vi "Animate Beer.vi"(10 "Type":enum16{"Lager", "Ale", "Guiness"}(ring)=enum."Guiness", 11 "Tilt":bool) -> ()   [LabVIEW 2011]
doc: "This shows teh animation of a beer being poured"
uses:
  <vilib>/vision/NI_Vision_Development_Module.lvlib
panel:
  out "Image 2":T1(plugin-control)
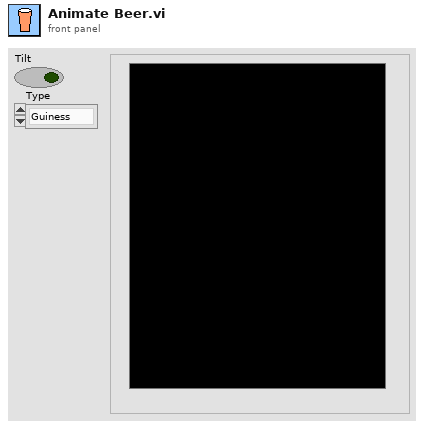
[diagram p1: front panel]
types:
  T1 = typedef "IMAQ Image.ctl" = refnum<image>
  T2 = typedef "Image Type" = u32
  T3 = cluster{"Red or Hue value":u8, "Green or Sat value":u8, "Blue or Luma or Val or Inten value":u8}
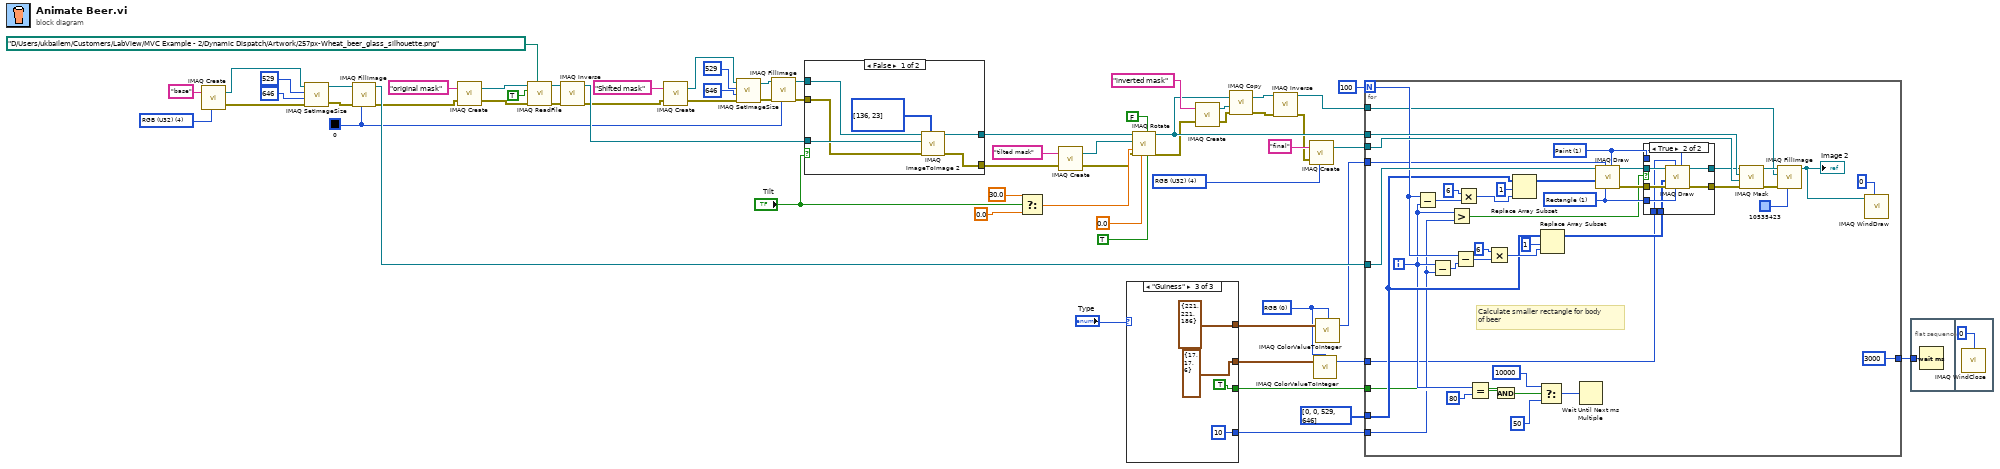
[diagram p0: block diagram]
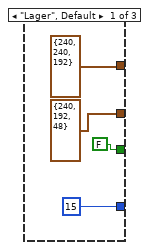
[diagram p2: hidden frame]
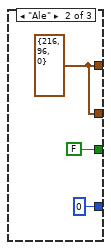
[diagram p3: hidden frame]
diagram:
  w18 = u16 0 items=["RGB", "HSL", "HSV", "HSI"] ("Color Mode")
  w16 = u32 0 ("Color Pixel Value")
  w43 = T2 4 items=["Grayscale (U8)", "Grayscale (I16)", "Grayscale (SGL)", "Complex (CSG)", "RGB (U32)", "HSL (U32)", "RGB (U64)", "Grayscale (U16)"] ("Image Type")
  w52 = T2 4 items=["Grayscale (U8)", "Grayscale (I16)", "Grayscale (SGL)", "Complex (CSG)", "RGB (U32)", "HSL (U32)", "RGB (U64)", "Grayscale (U16)"] ("Image Type")
  n1 = call "IMAQ Create"("Image Name"="base", "Image Type"=w52) -> ("New Image"=w51:T1, "error out"=w50:errorcluster)  [unwired: 3 in]
  n2 = call "IMAQ SetImageSize"("error in (no error)"=w50, "Y Resolution"=646, "X Resolution"=529, "Image"=w51) -> ("error out"=w47:errorcluster, "Image Out"=w48:T1)  [unwired: 1 in]
  n3 = call "IMAQ FillImage"("Color Pixel Value"=w16, "error in (no error)"=w47, "Image"=w48) -> ("error out"=w21:errorcluster, "Image Out"=w45:T1)  [unwired: 7 in]
  n4 = call "IMAQ Create"("Image Name"="original mask", "error in (no error)"=w21) -> ("New Image"=w62:T1, "error out"=w63:errorcluster)  [unwired: 3 in]
  n5 = call "IMAQ ReadFile"("File Path"=path "D:/Users/ukbailem/Customers/LabView/MVC Example - 2/Dynamic Dispatch/Artwork/257px-Wheat_beer_glass_silhouette.png" ("Path"), "error in (no error)"=w63, "Load Color Palette? (No)"=TRUE, "Image"=w62) -> ("error out"=w23:errorcluster, "Image Out"=w54:T1)  [unwired: 3 in, 3 out]
  n6 = call "IMAQ Inverse"("error in (no error)"=w23, "Image Src"=w54) -> ("error out"=w22:errorcluster, "Image Dst Out"=w28:T1)  [unwired: 8 in]
  n7 = call "IMAQ Create"("Image Name"="Shifted mask", "error in (no error)"=w22) -> ("New Image"=w33:T1, "error out"=w32:errorcluster)  [unwired: 3 in]
  n8 = call "IMAQ SetImageSize"("error in (no error)"=w32, "Y Resolution"=646, "X Resolution"=529, "Image"=w33) -> ("error out"=w31:errorcluster, "Image Out"=w30:T1)  [unwired: 1 in]
  n9 = call "IMAQ FillImage"("Color Pixel Value"=w16, "error in (no error)"=w31, "Image"=w30) -> ("error out"=w20:errorcluster, "Image Out"=w29:T1)  [unwired: 7 in]
  n10 = case shown="False" "Tilt" {
    tunnel: w29 -> [w70 _]
    tunnel: w28 -> [w69 w72]
    tunnel: [w68 w72] -> w27
    tunnel: w20 -> [w66 w71]
    tunnel: [w65 w71] -> w13
    frame False {
      n11 = call "IMAQ ImageToImage 2"("Offset Left/Top"=i32[] [136, 23], "error in (no error)"=w66, "Image Src (Small)"=w69, "Image Src (Large)"=w70) -> ("error out"=w65:errorcluster, "Image Dst Out"=w68:T1)  [unwired: 6 in]
    }
    frame True {
    }
  }
  n12 = Select(t=sgl 30.0 ("Angle (degrees)"), s="Tilt", f=sgl 0.0) -> (s? t:f=w38:sgl)
  n13 = call "IMAQ Create"("Image Name"="tilted mask", "error in (no error)"=w13) -> ("New Image"=w58:T1, "error out"=w3:errorcluster)  [unwired: 3 in]
  n14 = case shown="\"Guiness\"" "Type" {
    tunnel: [T3 {"Red or Hue value"=240, "Green or Sat value"=240, "Blue or Luma or Val or Inten value"=192} ("Color Value") w79 T3 {"Red or Hue value"=221, "Green or Sat value"=221, "Blue or Luma or Val or Inten value"=186} ("Color Value")] -> w24
    tunnel: [T3 {"Red or Hue value"=240, "Green or Sat value"=192, "Blue or Luma or Val or Inten value"=48} ("Color Value") w79 T3 {"Red or Hue value"=17, "Green or Sat value"=17, "Blue or Luma or Val or Inten value"=6} ("Color Value")] -> w15
    tunnel: [FALSE FALSE TRUE] -> w14
    tunnel: [15 ("y") 0 ("y") 10 ("y")] -> w7
    frame "Lager", Default {
    }
    frame "Ale" {
      w79 = T3 {"Red or Hue value"=216, "Green or Sat value"=96, "Blue or Luma or Val or Inten value"=0} ("Color Value")
    }
    frame "Guiness" {
    }
  }
  n15 = call "IMAQ Rotate"("Use Bilinear Interpolation"=TRUE, "Maintain Size"=FALSE, "Replace Value"=sgl 0.0, "error in (no error)"=w3, "Angle (degrees)"=w38, "Image Dst"=w58, "Image Src"=w27) -> ("error out"=w1:errorcluster, "Image Dst Out"=w11:T1)  [unwired: 3 in]
  n16 = call "IMAQ Create"("Image Name"="inverted mask", "error in (no error)"=w1) -> ("New Image"=w10:T1, "error out"=w2:errorcluster)  [unwired: 3 in]
  n17 = call "IMAQ Copy"("error in (no error)"=w2, "Image Dst"=w10, "Image Src"=w11) -> ("error out"=w5:errorcluster, "Image Dst Out"=w9:T1)  [unwired: 3 in]
  n18 = call "IMAQ Inverse"("error in (no error)"=w5, "Image Src"=w9) -> ("error out"=w4:errorcluster, "Image Dst Out"=w8:T1)  [unwired: 8 in]
  n19 = call "IMAQ Create"("Image Name"="final", "Image Type"=w43, "error in (no error)"=w4) -> ("New Image"=w40:T1)  [unwired: 2 in, 1 out]
  n20 = call "IMAQ ColorValueToInteger"("Color Value"=w15, "Color Mode"=w18) -> ("U32 value"=w17:u32)  [unwired: 3 in, 3 out]
  n21 = call "IMAQ ColorValueToInteger"("Color Value"=w24, "Color Mode"=w18) -> ("U32 value"=w25:u32)  [unwired: 3 in, 3 out]
  n22 = for {
    N: 100 -> [w116]
    tunnel: w45 -> [w124]
    tunnel: i32[] [0, 0, 529, 646] ("Coordinates") -> [w106]
    tunnel: w11 -> [w120]
    tunnel: w40 -> [w119]
    tunnel: w25 -> [w85]
    tunnel: w17 -> [w84]
    tunnel: w14 -> [w94]
    tunnel: w8 -> [w92]
    tunnel: w7 -> [w89]
    tunnel: [u32 3000 ("t")] -> w6
    i -> [w96]
    w110 = u16 1 items=["Frame", "Paint", "Invert Frame", "Invert Paint"] ("Draw Mode")
    w109 = u16 1 items=["Line", "Rectangle", "Oval"] ("Shape to draw")
    # "Calculate smaller rectangle for body\nof beer"
    n23 = Subtract(x=w116, y=w96) -> (x-y=w122:i32)
    n24 = Subtract(x=w96, y=w89) -> (x-y=w117:i32)
    n25 = Greater?(x=w96, y=w89) -> (0:w104:bool)
    n26 = Subtract(x=w116, y=w117) -> (x-y=w115:i32)
    n27 = Multiply(x=6, y=w122) -> (x*y=w107:i32)
    n28 = Equal?(x=w96, y=80) -> (x = y?=w100:bool)
    n29 = Multiply(x=6, y=w115) -> (x*y=w108:i32)
    n30 = And(x=w100, y=w94) -> (x .and. y?=w95:bool)
    n31 = Replace Array Subset(array=w106, new element=w107, index=1) -> (w103:i32[])
    n32 = Select(t=u32 10000, s=w95, f=u32 50 ("millisecond multiple")) -> (s? t:f=w97:u32)
    n33 = Replace Array Subset(array=w106, new element=w108, index=1) -> (w102:i32[])
    n34 = Wait Until Next ms Multiple(millisecond multiple=w97) -> ()  [unwired: 1 out]
    n35 = call "IMAQ Draw"("Draw Mode"=w110, "Shape to draw"=w109, "Pixel Color"=w85, "Coordinates"=w103, "Image Src"=w124) -> ("error out"=w114:errorcluster, "Image Dst Out"=w111:T1)  [unwired: 5 in]
    n36 = case shown="True" w104 {
      tunnel: w114 -> [w125 w134]
      tunnel: [w125 w133] -> w113
      tunnel: [w126 w132] -> w112
      tunnel: w111 -> [w126 w131]
      tunnel: w110 -> [_ w130]
      tunnel: w109 -> [_ w129]
      tunnel: w102 -> [_ w128]
      tunnel: w84 -> [_ w127]
      frame False {
      }
      frame True {
        n37 = call "IMAQ Draw"("Draw Mode"=w130, "Shape to draw"=w129, "Pixel Color"=w127, "error in (no error)"=w134, "Coordinates"=w128, "Image Src"=w131) -> ("error out"=w133:errorcluster, "Image Dst Out"=w132:T1)  [unwired: 4 in]
      }
    }
    n38 = call "IMAQ Mask"("error in (no error)"=w113, "Image Dst"=w119, "Image Mask"=w120, "Image Src"=w112) -> ("error out"=w91:errorcluster, "Image Dst Out"=w93:T1)  [unwired: 1 in]
    n39 = call "IMAQ FillImage"("Color Pixel Value"=u32 10535423, "error in (no error)"=w91, "Image Mask"=w92, "Image"=w93) -> ("Image Out"=w87:T1)  [unwired: 6 in, 1 out]
    "Image 2" <- w87
    n40 = call "IMAQ WindDraw"("Window Number (0...15)"=0, "Image"=w87) -> ()  [unwired: 8 in, 2 out]
  }
  n41 = flat-sequence {
    tunnel: w6 -> [w135]
    frame #0 {
      n42 = Wait (ms)(milliseconds to wait=w135) -> ()  [unwired: 1 out]
    }
    frame #1 {
      n43 = call "IMAQ WindClose"("Window Number (0...15)"=0) -> ()  [unwired: 5 in, 1 out]
    }
  }
